vi "1D_index_to_pixel_XY.vi"(2 "ID Index":i32, 3 "Image Height":i32) -> (0 "Y":i32, 1 "X":i32)   [LabVIEW 2019]
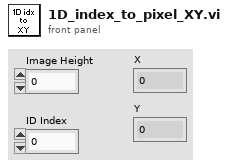
[diagram p1: front panel]
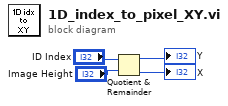
[diagram p0: block diagram]
diagram:
  n1 = Quotient & Remainder(x="ID Index", y="Image Height") -> (x-y*floor(x/y)=→"Y":i32, floor(x/y)=→"X":i32)
